vi "New Report Action.vi"(8 "error in":errorcluster, 11 "M_Butt in":refnum<class "Manual_Buttons.lvclass">) -> (0 "error out":errorcluster, 3 "M_Butt out":refnum<class "Manual_Buttons.lvclass">)   [LabVIEW 2023, in "Manual_Buttons.lvlib" / "Manual_Buttons.lvclass"]
doc: "Send Create new report event to report generator by closing the current report and creating a new one."
uses:
  Project/Manual_Buttons.lvclass
  C:/Users/Public/Documents/Development/builds/Engine/Engine.lvlibp/Project/Engine.lvclass
  builds/Engine/Engine.lvlibp/Accessors/Read Report Queue.vi
  builds/Tools/QDMH.lvlibp/QDMH.lvclass
  builds/Engine/Engine.lvlibp/Project/Engine.lvclass
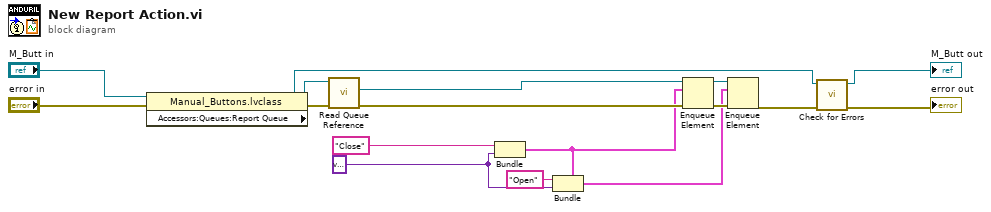
[diagram p0: block diagram]
diagram:
  w6 = variant
  n1 = property class="Manual_Buttons.lvclass"(reference="M_Butt in", error in="error in") -> (reference out=w3:refnum<class "Manual_Buttons.lvclass">, error out=w12:errorcluster, "Accessors:Queues:Report Queue"=w14:refnum<class "QDMH.lvclass">)
  n2 = call "Read Queue Reference.vi"("error in"=w12, "QDMH in"=w14) -> ("error out"=w11:errorcluster, "Queue Reference"=w13:refnum<queue>)  [unwired: 7 in, 1 out]
  n3 = Bundle("Close", w6) -> (w10:cluster{string, variant})  [unwired: 1 in]
  n4 = Bundle(cluster=w10, "Open", w6) -> (w7:cluster{string, variant})
  n5 = Enqueue Element(queue=w13, element=w10, error in (no error)=w11) -> (queue out=w8:refnum<queue>, error out=w9:errorcluster)  [unwired: 1 in, 1 out]
  n6 = Enqueue Element(queue=w8, element=w7, error in (no error)=w9) -> (error out=w4:errorcluster)  [unwired: 1 in, 2 out]
  n7 = call "Check for Errors.vi"("error in"=w4, "Engine in"=w3) -> ("error out"=→"error out":errorcluster, "Engine out"=→"M_Butt out":refnum<class "Manual_Buttons.lvclass">)  [unwired: 8 in]
